vi "画圆复刻.vi"() -> ()   [LabVIEW 2018]
panel:
  in  "颜色盒":u32(colorbox)
  in  "是否填充":bool
  out "画布":picture
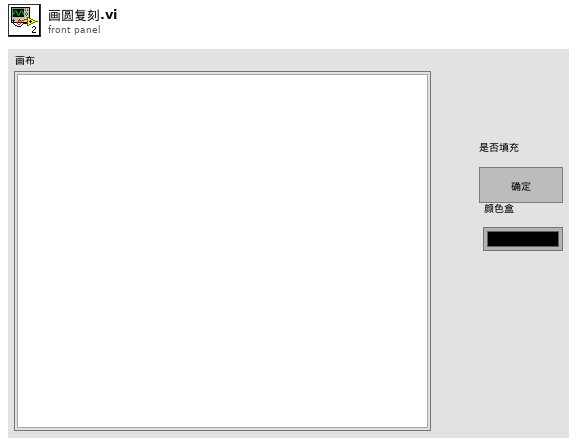
[diagram p1: front panel]
types:
  T1 = typedef "LVMouseTypeDef.ctl" = cluster{"Mouse Position":cluster{"X":i32, "Y":i32}, "Mouse Modifiers":cluster{"Button Down":bool, "Shift Mod":bool, "Menu Mod":bool, "Option Mod":bool}}
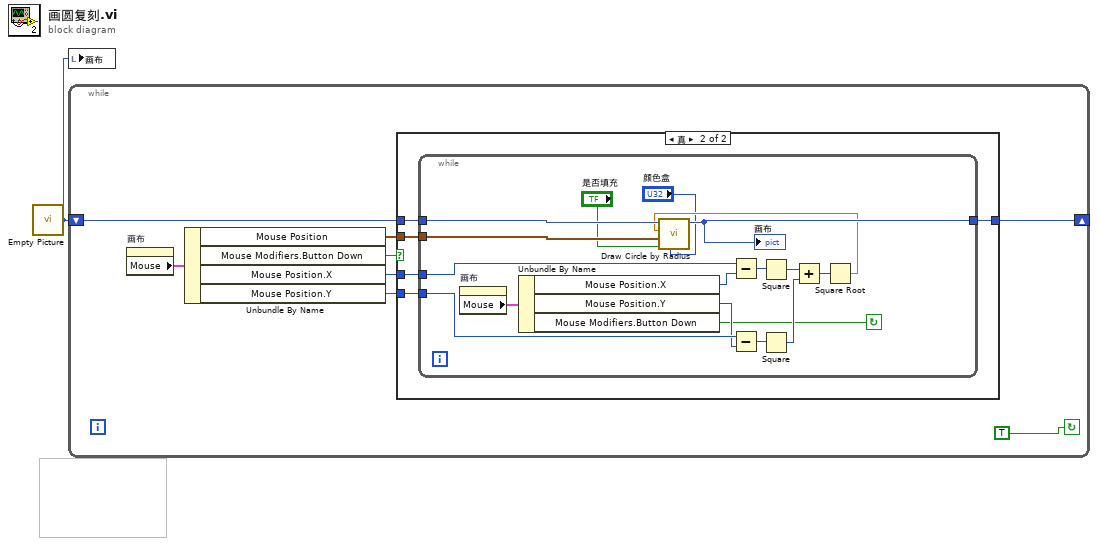
[diagram p0: block diagram]
diagram:
  n1 = call "Empty Picture"() -> ("empty picture"=w1:picture)
  n2 = local write "画布"(w1) -> ()
  n3 = while {
    shift-right: [w5] -> _
    shift-left: w1 -> [w6]
    stop <- TRUE continue-if-true
    n4 = property on="画布" class="Pict"() -> ("Mouse"=w9:T1)  [unwired: 2 in, 2 out]
    n5 = Unbundle By Name(w9) -> ("Mouse Position"=w7:cluster{"X":i32, "Y":i32}, "Mouse Modifiers.Button Down"=w8:bool, "Mouse Position.X"=w4:i32, "Mouse Position.Y"=w3:i32)
    n6 = case shown="真" w8 {
      tunnel: w7 -> [_ w14]
      tunnel: w6 -> [w10 w15]
      tunnel: [w10 w13] -> w5
      tunnel: w4 -> [_ w12]
      tunnel: w3 -> [_ w11]
      frame False {
      }
      frame True {
        n7 = while {
          tunnel: w15 -> [w32]
          tunnel: w14 -> [w30]
          tunnel: [w29] -> w13
          tunnel: w12 -> [w27]
          tunnel: w11 -> [w23]
          stop <- w16 continue-if-true
          n8 = property on="画布" class="Pict"() -> ("Mouse"=w31:T1)  [unwired: 2 in, 2 out]
          n9 = Unbundle By Name(w31) -> ("Mouse Position.X"=w26:i32, "Mouse Position.Y"=w22:i32, "Mouse Modifiers.Button Down"=w16:bool)
          n10 = Subtract(x=w27, y=w26) -> (x-y=w25:i32)
          n11 = Subtract(x=w23, y=w22) -> (x-y=w21:i32)
          n12 = Square(x=w25) -> (x^2=w24:i32)
          n13 = Square(x=w21) -> (x^2=w20:i32)
          n14 = Add(x=w24, y=w20) -> (x+y=w28:i32)
          n15 = Square Root(x=w28) -> (sqrt(x)=w19:dbl)
          n16 = call <vilib>:"Draw Circle by Radius.vi"("color(black)"="颜色盒", "fill?(F)"="是否填充", "pixel center"=w30, "radius"=w19, "picture"=w32) -> ("new picture"=w29:picture)  [unwired: 6 in]
          "画布" <- w29
        }
      }
    }
  }
